vi "checkBeginEnemyPossesionAtOurField.vi"(8 "error in (no error)":errorcluster, 10 "Game":refnum<class "Game.lvclass">, 11 "EnemyPossessionAtOurFieldPlay in":refnum<class "EnemyPossessionAtOurFieldPlay.lvclass">) -> (0 "error out":errorcluster, 2 "Begin?":bool, 3 "EnemyPossessionAtOurFieldPlay out":refnum<class "EnemyPossessionAtOurFieldPlay.lvclass">)   [LabVIEW 2023, in "EnemyPossessionAtOurFieldPlay.lvclass"]
uses:
  EnemyPossessionAtOurFieldPlay.lvclass
  Game_class/Game.lvclass
  Game_class/Game.lvclass/Game.ctl
  Events_class/Events.lvclass/Events.ctl
  Object_class/Object.lvclass/Object.ctl
  Game_class/Read Referee.vi
  Game_class/Read EventsRef.vi
  Game_class/Read BallRef.vi
  Object_class/Read x.vi
  Events_class/Read enemy_ball_possesion.vi
  Ball_class/Ball.lvclass
  Referee_class/Referee.lvclass
  Events_class/Events.lvclass
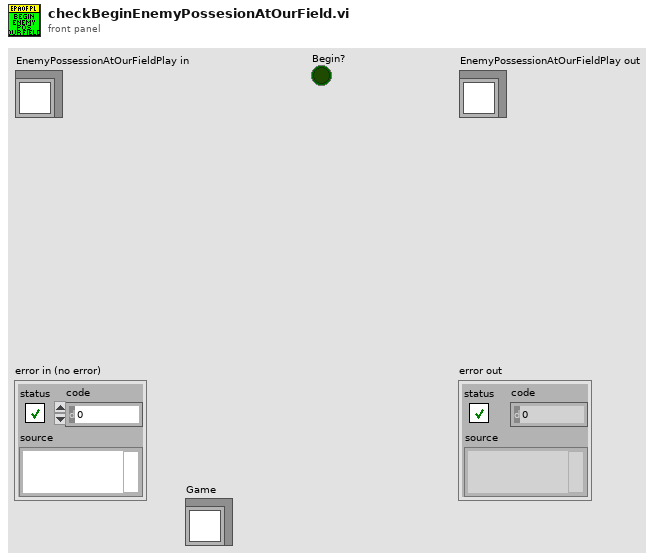
[diagram p1: front panel]
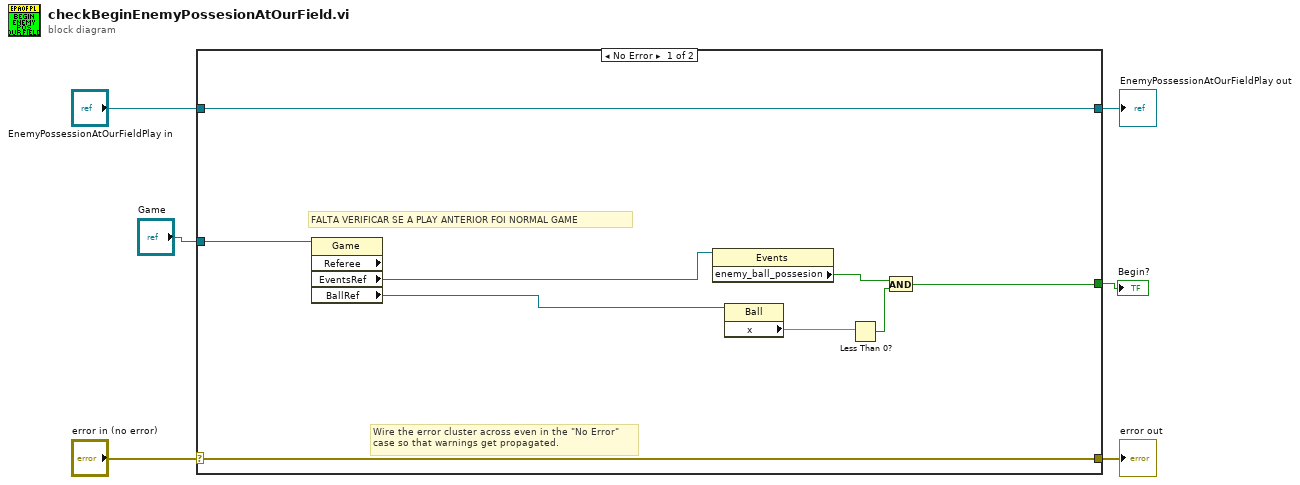
[diagram p0: block diagram]
diagram:
  n1 = case shown="No Error" "error in (no error)" {
    selector: "error in (no error)" -> [w14 w17]
    tunnel: [w14 w17] -> w5
    tunnel: [w15 w16] -> w3
    tunnel: "EnemyPossessionAtOurFieldPlay in" -> [w15 w16]
    tunnel: "Game" -> [w9 _]
    tunnel: [w8 _] -> w1
    frame No Error {
      # "FALTA VERIFICAR SE A PLAY ANTERIOR FOI NORMAL GAME"
      # "Wire the error cluster across even in the \"No Error\"\ncase so that warnings get propagated."
      n2 = property class="Game" props=["Referee", "EventsRef", "BallRef"](reference=w9) -> ("EventsRef"=w13:refnum<class "Events.lvclass">, "BallRef"=w12:refnum<class "Ball.lvclass">)  [unwired: 1 in, 3 out]
      n3 = property class="Events"(reference=w13) -> ("enemy_ball_possesion"=w7:bool)  [unwired: 1 in, 2 out]
      n4 = property class="Ball"(reference=w12) -> ("x"=w11:dbl)  [unwired: 1 in, 2 out]
      n5 = Less Than 0?(x=w11) -> (x < 0?=w10:bool)
      n6 = And(x=w7, y=w10) -> (x .and. y?=w8:bool)
    }
    frame Error {
    }
  }
  "error out" <- w5
  "EnemyPossessionAtOurFieldPlay out" <- w3
  "Begin?" <- w1
